vi "Read_and_Crypt_a_File.vi"(8 "error in (no error)":errorcluster, 9 "name of File":string, 10 "name of Folder":string, 11 "object in":refnum<class "Crypter.lvclass">) -> (0 "error out":errorcluster, 2 "Encrypted text":string, 3 "object out":refnum<class "Crypter.lvclass">, 5 "Crypting,,,,,,":path)   [LabVIEW 2016, in "Crypter.lvclass"]
uses:
  Crypter.lvclass
  Crypter.lvclass/Crypter.ctl
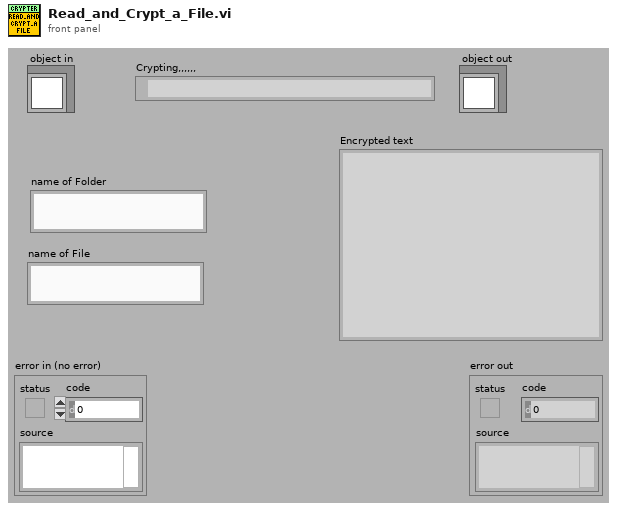
[diagram p1: front panel]
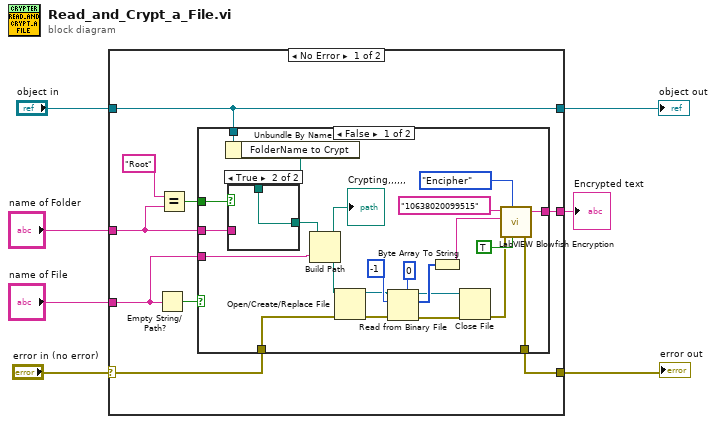
[diagram p0: block diagram]
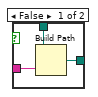
[diagram p2: hidden frame]
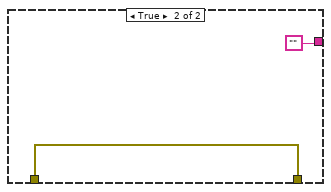
[diagram p3: hidden frame]
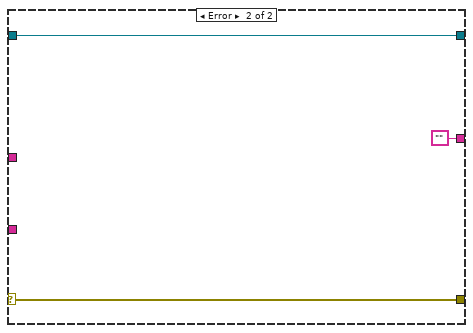
[diagram p4: hidden frame]
diagram:
  n1 = case shown="No Error" "error in (no error)" {
    selector: "error in (no error)" -> [w15 w47]
    tunnel: [w14 w47] -> w6
    tunnel: [w16 w46] -> w4
    tunnel: "object in" -> [w16 w46]
    tunnel: [w13 "" ("Output text")] -> w3
    tunnel: "name of Folder" -> [w11 _]
    tunnel: "name of File" -> [w8 _]
    frame No Error {
      n2 = Empty String/Path?(string/path=w8) -> (empty?=w9:bool)
      n3 = Equal?(x="Root", y=w11) -> (x = y?=w12:bool)
      n4 = case shown="False" w9 {
        tunnel: w16 -> [w38 _]
        tunnel: w15 -> [w32 w44]
        tunnel: [w31 w44] -> w14
        tunnel: [w30 ""] -> w13
        tunnel: w8 -> [w28 _]
        tunnel: w12 -> [w27 _]
        tunnel: w11 -> [w26 _]
        frame False {
          n5 = Unbundle By Name(w38) -> ("FolderName to Crypt"=w34:path)
          n6 = case shown="True" w27 {
            tunnel: [w41 w42] -> w35
            tunnel: w34 -> [w40 w42]
            tunnel: w26 -> [w39 _]
            frame False {
              n7 = Build Path(base path=w40, name or relative path=w39) -> (appended path=w41:path)
            }
            frame True {
            }
          }
          n8 = Build Path(base path=w35, name or relative path=w28) -> (appended path=w29:path)
          "Crypting,,,,,," <- w29
          n9 = Open/Create/Replace File(file path (use dialog)=w29, error in=w32) -> (refnum out=w22:refnum<file>, error out=w21:errorcluster)  [unwired: 4 in, 1 out]
          n10 = Read from Binary File(5:u8 0, 8:w21, 10:-1 ("count (1)"), 11:w22) -> (0:w20:errorcluster, 2:w23:u8[], 3:w19:refnum<file>)  [unwired: 2 in, 1 out]
          n11 = Byte Array To String(unsigned byte array=w23) -> (string=w18:string)
          n12 = Close File(refnum=w19, error in=w20) -> (error out=w33:errorcluster)  [unwired: 1 out]
          n13 = call "LabVIEW Blowfish Encryption.vi"("Password"="10638020099515", "Enc/Dec"=enum16{"Encipher", "Decipher"}."Encipher", "Input Text"=w18, "Output As ASCII\nfor email Transmission"=TRUE ("Output As ASCII\nfor email Transmission"), "error in (no error)"=w33) -> ("Output text"=w30:string, "error out"=w31:errorcluster)  [unwired: 1 in, 1 out]
        }
        frame True {
        }
      }
    }
    frame Error {
    }
  }
  "error out" <- w6
  "object out" <- w4
  "Encrypted text" <- w3
